vi "Evaluate Case Status.vi"(10 "Results":T1[](array[typedef]), 11 "Current":T2) -> (3 "Status":T2=enum."Passed")   [LabVIEW 2020, in "LUnit Test Suite.lvclass"]
uses:
  LUnit Test Suite.lvclass
  LUnit Test Suite.lvclass/LUnit Test Suite.ctl
  Result/Status.ctl
  Result/Result.lvlib
  Result/Type.ctl
  Result/Result.ctl
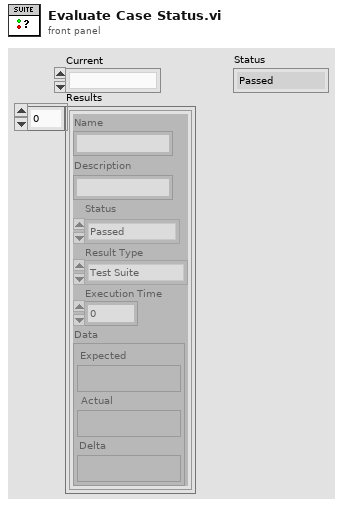
[diagram p1: front panel]
types:
  T1 = typedef "Result.lvlib/Result.ctl" = cluster{"Name":string, "Description":string, "Status":T2, "Result Type":T3, "Execution Time":dbl, "Data":cluster{"Expected":variant, "Actual":variant, "Delta":variant}}
  T2 = typedef "Result.lvlib/Status.ctl" = enum16{"", "Passed", "Failed", "Error", "Skipped", "Setup Error", "Broken", "Teardown Error"}
  T3 = typedef "Result.lvlib/Type.ctl" = enum16{"Test Case", "Test Suite", "Test Run", "Pass", "Fail", "Skip", "Pass if", "Fail if", "Pass if Error", "Fail if Error", "Pass if Equal", "Fail if Equal"}
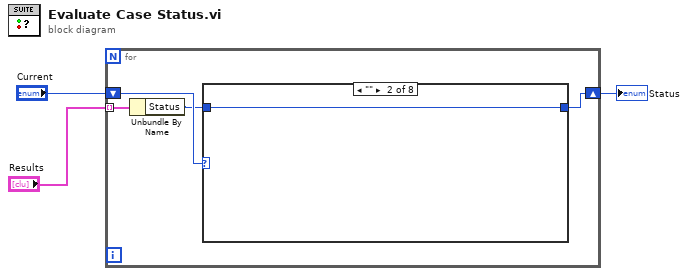
[diagram p0: block diagram]
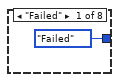
[diagram p3: hidden frame]
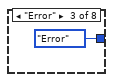
[diagram p4: hidden frame]
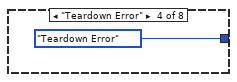
[diagram p5: hidden frame]
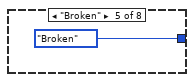
[diagram p6: hidden frame]
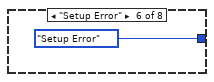
[diagram p7: hidden frame]
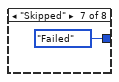
[diagram p8: hidden frame]
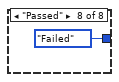
[diagram p9: hidden frame]
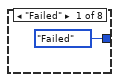
[diagram p11: hidden frame]
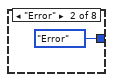
[diagram p12: hidden frame]
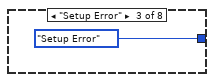
[diagram p13: hidden frame]
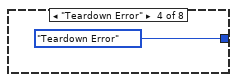
[diagram p14: hidden frame]
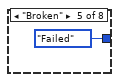
[diagram p15: hidden frame]
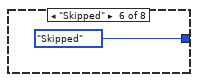
[diagram p16: hidden frame]
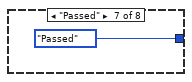
[diagram p17: hidden frame]
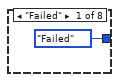
[diagram p19: hidden frame]
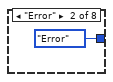
[diagram p20: hidden frame]
diagram:
  n1 = for {
    shift-right: [w6] -> w3
    shift-left: "Current" -> [w7]
    tunnel: "Results" -> [w5] mode=indexing
    n2 = Unbundle By Name(w5) -> ("Status"=w4:T2)
    n3 = case shown="\"\"" w7 {
      selector: w7 -> [w8 _ w20 w31 _ _ _ _]
      tunnel: w4 -> [w10 w19 w22 w33 _ _ w44 w48]
      tunnel: [w9 w19 w21 w32 Status."Error" ("Merged Status") Status."Setup Error" ("Merged Status") w45 w48] -> w6
      frame "Failed" {
        n4 = case shown="\"\"" w10 {
          tunnel: [Status."Failed" ("Merged Status") w12 Status."Error" ("Merged Status") Status."Teardown Error" ("Merged Status") Status."Broken" ("Merged Status") Status."Setup Error" ("Merged Status") Status."Failed" ("Merged Status") Status."Failed" ("Merged Status")] -> w9
          tunnel: w8 -> [_ w12 _ _ _ _ _ _]
          frame "Failed" {
          }
          frame "" {
          }
          frame "Error" {
          }
          frame "Teardown Error" {
          }
          frame "Broken" {
          }
          frame "Setup Error" {
          }
          frame "Skipped" {
          }
          frame "Passed" {
          }
        }
      }
      frame "" {
      }
      frame "Skipped" {
        n5 = case shown="\"\"" w22 {
          tunnel: [Status."Failed" ("Merged Status") Status."Error" ("Merged Status") Status."Setup Error" ("Merged Status") Status."Teardown Error" ("Merged Status") Status."Failed" ("Merged Status") Status."Skipped" ("Merged Status") Status."Passed" ("Merged Status") w30] -> w21
          tunnel: w20 -> [_ _ _ _ _ _ _ w30]
          frame "Failed" {
          }
          frame "Error" {
          }
          frame "Setup Error" {
          }
          frame "Teardown Error" {
          }
          frame "Broken" {
          }
          frame "Skipped" {
          }
          frame "Passed" {
          }
          frame "" {
          }
        }
      }
      frame "Passed" {
        n6 = case shown="\"\"" w33 {
          tunnel: [Status."Failed" ("Merged Status") Status."Error" ("Merged Status") Status."Setup Error" ("Merged Status") Status."Failed" ("Merged Status") Status."Teardown Error" ("Merged Status") Status."Passed" ("Merged Status") w40 Status."Passed" ("Merged Status")] -> w32
          tunnel: w31 -> [_ _ _ _ _ _ w40 _]
          frame "Failed" {
          }
          frame "Error" {
          }
          frame "Setup Error" {
          }
          frame "Broken" {
          }
          frame "Teardown Error" {
          }
          frame "Skipped" {
          }
          frame "" {
          }
          frame "Passed" {
          }
        }
      }
      frame "Error" {
      }
      frame "Setup Error" {
      }
      frame "Teardown Error" {
        n7 = case shown="\"Error\", \"Setup Error\", \"Broken\"" w44 {
          selector: w44 -> [_ w47]
          tunnel: [Status."Teardown Error" ("Merged Status") w47] -> w45
          frame Default {
          }
          frame "Error", "Setup Error", "Broken" {
          }
        }
      }
      frame "Broken" {
      }
    }
  }
  "Status" <- w3
